vi "LV-SubVI-Acquiris.vi"(0 "file path":path, 1 "error in":errorcluster) -> (2 "path":path, 3 "waveform":i8[](array[numeric]), 4 "error out":errorcluster)   [LabVIEW 2010]
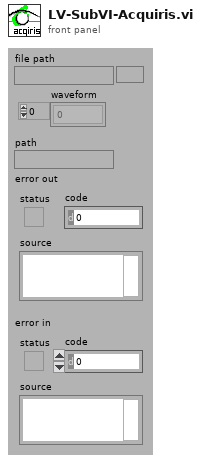
[diagram p1: front panel]
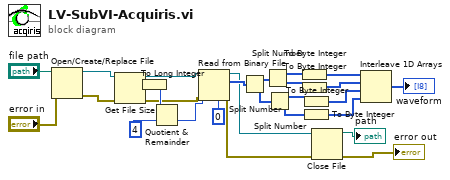
[diagram p0: block diagram]
diagram:
  n1 = Open/Create/Replace File(file path (use dialog)="file path", error in="error in") -> (refnum out=w26:refnum<file>, error out=w10:errorcluster)  [unwired: 4 in, 1 out]
  n2 = Get File Size(file=w26, error in=w10) -> (refnum out=w12:refnum<file>, size (in bytes)=w1:i64, 0:w9:errorcluster)
  n3 = To Long Integer(number=w1) -> (32bit integer=w15:i32)
  n4 = Quotient & Remainder(x=w15, y=4) -> (floor(x/y)=w13:i32)  [unwired: 1 out]
  n5 = Read from Binary File(5:0 ("byte stream type"), 8:w9, 10:w13, 11:w12) -> (0:w7:errorcluster, 2:w27:i32[], 3:w8:refnum<file>)  [unwired: 2 in, 1 out]
  n6 = Split Number(x=w27) -> (hi(x)=w25:u16[], lo(x)=w22:u16[])
  n7 = Split Number(x=w25) -> (hi(x)=w24:u8[], lo(x)=w23:u8[])
  n8 = Split Number(x=w22) -> (hi(x)=w20:u8[], lo(x)=w21:u8[])
  n9 = To Byte Integer(number=w24) -> (8bit integer=w19:i8[])
  n10 = To Byte Integer(number=w23) -> (8bit integer=w18:i8[])
  n11 = To Byte Integer(number=w20) -> (8bit integer=w17:i8[])
  n12 = To Byte Integer(number=w21) -> (8bit integer=w16:i8[])
  n13 = Close File(refnum=w8, error in=w7) -> (path=→"path":path, error out=→"error out":errorcluster)
  n14 = Interleave 1D Arrays(w19, w18, w17, w16) -> (→"waveform":i8[])
